vi "GyroReset_Simulation_Global.vi"(0 "menu":enum16{"set", "get", "delete"}(ring)=enum."get", 5 "Gyro Channel":T1=enum."AI 1", 7 "reset in":bool, 11 "error in (no error)":errorcluster) -> (8 "reset out":bool, 15 "error out":errorcluster)   [LabVIEW 2017]
doc: "This is used to set and get whether a gyro reset has been issued.\n\nThis software is licensed. Open the labview\\readme\\WPI Robotics Library Open Source License.txt file for more information."
uses:
  <vilib>/Rock Robotics/SystemInterfaces/AI/FPGA_AIGyroChannel.ctl
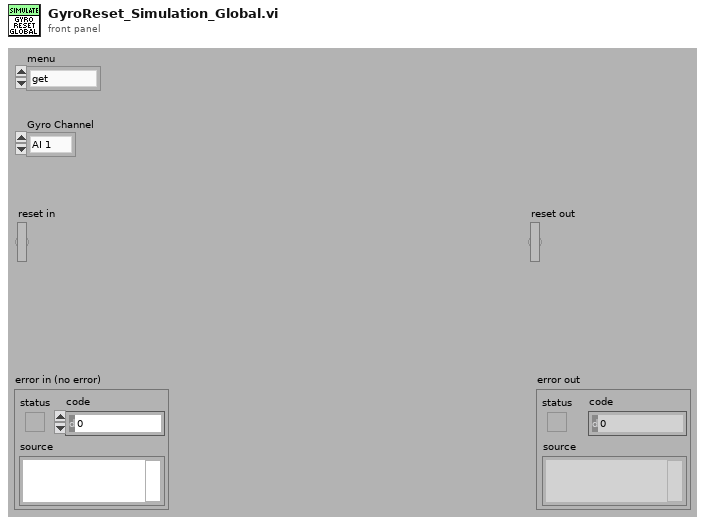
[diagram p1: front panel]
types:
  T1 = typedef "FPGA_AIGyroChannel.ctl" = enum8{"AI 0", "AI 1", "Invalid"}
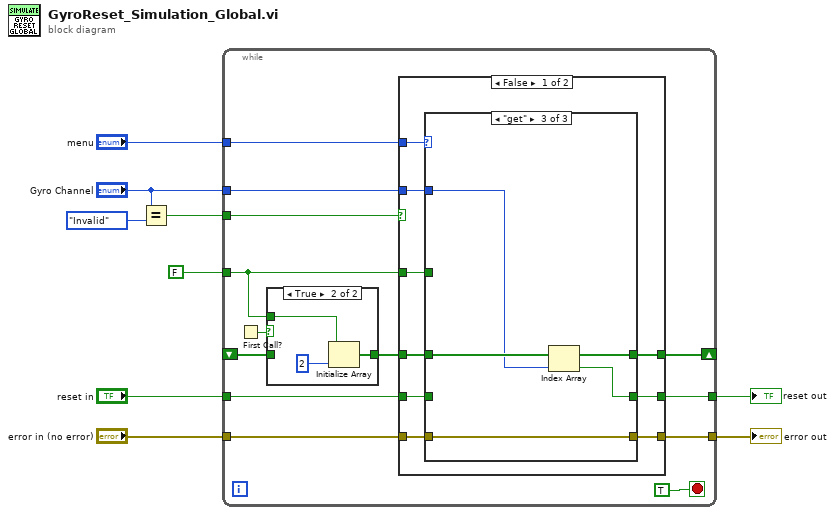
[diagram p0: block diagram]
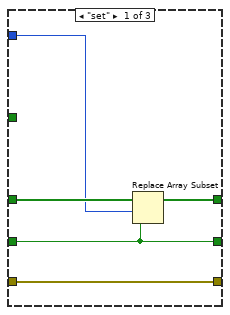
[diagram p2: hidden frame]
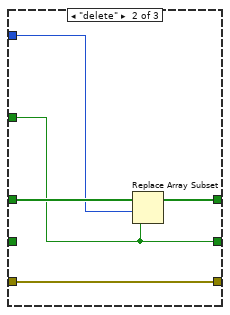
[diagram p3: hidden frame]
diagram:
  n1 = Equal?(x="Gyro Channel", y=FPGA_AIGyroChannel."Invalid" ("Encoder Index")) -> (x = y?=w5:bool)
  n2 = while {
    tunnel: "reset in" -> [w22]
    tunnel: "error in (no error)" -> [w18]
    shift-right: [w21] -> _
    shift-left: _ -> [w13]
    tunnel: [w20] -> w2
    tunnel: "menu" -> [w19]
    tunnel: [w17] -> w8
    tunnel: "Gyro Channel" -> [w12]
    tunnel: w5 -> [w11]
    tunnel: FALSE -> [w10]
    stop <- TRUE stop-if-true
    n3 = First Call?() -> (First Call?: T/F=w15:bool)
    n4 = case shown="True" w15 {
      tunnel: [w49 w51] -> w14
      tunnel: w13 -> [w49 _]
      tunnel: w10 -> [_ w50]
      frame False {
      }
      frame True {
        n5 = Initialize Array(w50, 2 ("dimension size")) -> (w51:bool[])
      }
    }
    n6 = case shown="False" w11 {
      tunnel: w22 -> [w31 _]
      tunnel: [w30 w48] -> w21
      tunnel: [w29 w46] -> w20
      tunnel: w19 -> [w28 _]
      tunnel: w18 -> [w27 w47]
      tunnel: [w26 w47] -> w17
      tunnel: w14 -> [w25 w48]
      tunnel: w12 -> [w24 _]
      tunnel: w10 -> [w23 w46]
      frame False {
        n7 = case shown="\"get\"" w28 {
          tunnel: w31 -> [w34 _ _]
          tunnel: [w35 w40 w45] -> w30
          tunnel: w25 -> [w36 w41 w45]
          tunnel: [w34 w38 w44] -> w29
          tunnel: [w33 w39 w43] -> w26
          tunnel: w27 -> [w33 w39 w43]
          tunnel: w24 -> [w32 w37 w42]
          tunnel: w23 -> [_ w38 _]
          frame "set" {
            n8 = Replace Array Subset(array=w36, new element=w34, index=w32) -> (w35:bool[])
          }
          frame "delete" {
            n9 = Replace Array Subset(array=w41, new element=w38, index=w37) -> (w40:bool[])
          }
          frame "get" {
            n10 = Index Array(array=w45, index=w42) -> (element=w44:bool)
          }
        }
      }
      frame True {
        # "Do nothing if channel is Invalid."
      }
    }
  }
  "error out" <- w8
  "reset out" <- w2
